vi "2D_Plot.ly_Ex.vi"() -> ()   [LabVIEW 2025]
doc: "Demonstratese how to plot an array with timebase to Plot.ly."
uses:
  <vilib>/Foerster.tech/LabPlot.ly/LabPlot.ly/Typdef/graphSettings.ctl
  <vilib>/Foerster.tech/LabPlot.ly/LabPlot.ly/Typdef/mode.ctl
  <vilib>/Foerster.tech/LabPlot.ly/LabPlot.ly/Typdef/line.ctl
  <vilib>/Foerster.tech/LabPlot.ly/LabPlot.ly/Typdef/dash.ctl
  <vilib>/Analysis/1siggen.llb/Ramp Pattern by Samples.vi
  <vilib>/Analysis/NI_AALBase.lvlib
  <vilib>/Foerster.tech/LabPlot.ly/LabPlot.ly/LabPlot.ly.lvlib
panel:
  out "File Path out":path
  out "Execution Time[ms]":u32
  in  "cycles":dbl=5.0 format="%0.2f"
  in  "Call Setup":bool
  in  "graphSettings":T1={"mode"=enum."lines+markers", "line"={"color"=44543, "width"=2, "dash"=enum."solid"}}
  in  "File Path Control(empty: only show graph)":path
  in  "Reduction(0: No Reduction)":i32
  in  "amplitude":dbl=5.0 format="%0.2f"
  in  "samples":i32=50000
  out "XY Graph":T5(graph)
  # "Sinewave Settings"
  # "Call asynchronously to not hold up your program"
  # "This Program demonstrates how to print a 2D Array consisting of timebase and data to Plot.ly\n\nYou can output the plot to browser without saving it by leaving File Path empty or save the html file by selecting a path.\n\nSince Plot.ly stores the data in the html, plots of >200k points become slow to open. It's recommended you use the built-in Reduction to reduce your dataset."
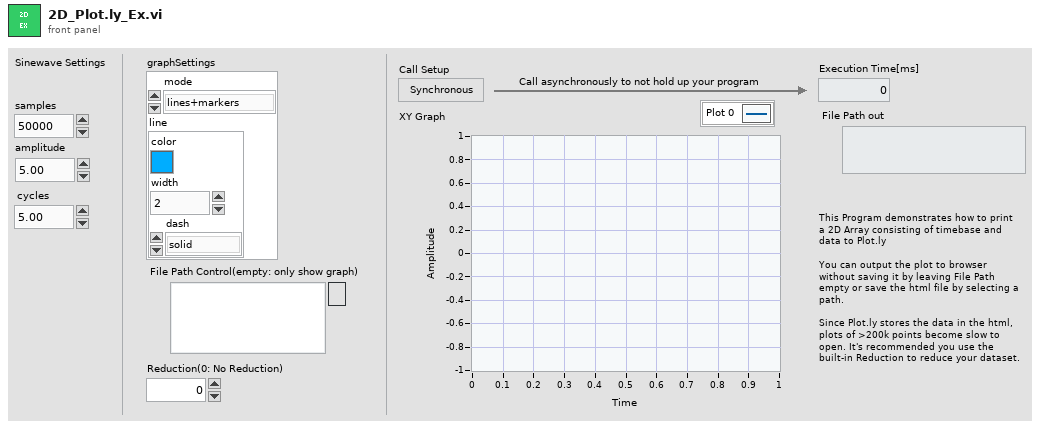
[diagram p1: front panel]
types:
  T1 = typedef "LabPlot.ly.lvlib/graphSettings.ctl" = cluster{"mode":T2, "line":T3}
  T2 = typedef "LabPlot.ly.lvlib/mode.ctl" = enum16{"lines", "markers", "text", "lines+markers", "markers+text", "lines+text", "lines+markers+text"}
  T3 = typedef "LabPlot.ly.lvlib/line.ctl" = cluster{"color":u32, "width":i32, "dash":T4}
  T4 = typedef "LabPlot.ly.lvlib/dash.ctl" = enum16{"solid", "dot", "dash", "longdash", "dashdot", "longdashdot"}
  T5 = cluster{"Ramp Pattern":dbl[], "Sinusoidal Pattern":dbl[]}
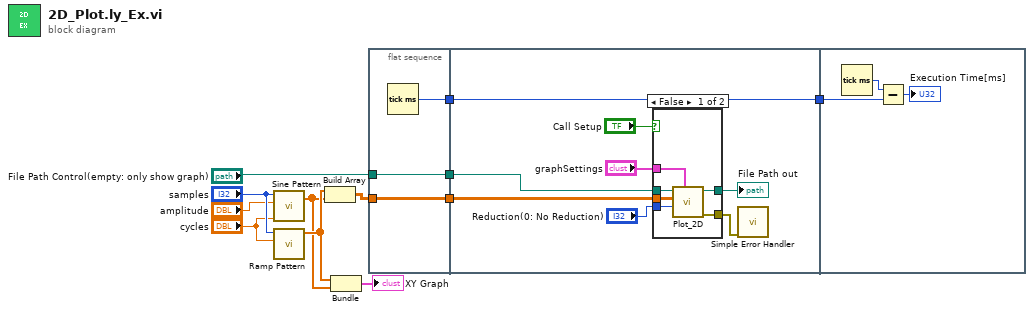
[diagram p0: block diagram]
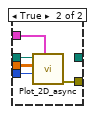
[diagram p2: hidden frame]
diagram:
  n1 = call <vilib>:"Sine Pattern.vi"("cycles"="cycles", "amplitude"="amplitude", "samples"="samples") -> ("Sinusoidal Pattern"=w6:dbl[])  [unwired: 1 in, 1 out]
  n2 = call-poly <vilib>:"Ramp Pattern.vi"("end"="cycles", "samples"="samples") -> ("Ramp Pattern"=w7:dbl[])  [unwired: 8 in, 1 out]
  n3 = Build Array(w7, w6) -> (w8:dbl[][])
  n4 = Bundle("Ramp Pattern"=w7, "Sinusoidal Pattern"=w6) -> (→"XY Graph":T5)  [unwired: 1 in]
  n5 = flat-sequence {
    tunnel: "File Path Control(empty: only show graph)" -> [w15]
    tunnel: [w15] -> w12
    tunnel: [w14] -> w11
    tunnel: w8 -> [w13]
    tunnel: [w13] -> w9
    tunnel: w12 -> [w23]
    tunnel: w11 -> [w22]
    tunnel: [w22] -> w10
    tunnel: w9 -> [w21]
    tunnel: w10 -> [w36]
    frame #0 {
      n6 = Tick Count (ms)() -> (millisecond timer value=w14:u32)
    }
    frame #1 {
      n7 = case shown="False" "Call Setup" {
        tunnel: "Reduction(0: No Reduction)" -> [w29 w32]
        tunnel: w23 -> [w28 w34]
        tunnel: "graphSettings" -> [w24 w33]
        tunnel: [w27 w31] -> w19
        tunnel: [w26 _] -> w20
        tunnel: w21 -> [w25 w30]
        frame False {
          n8 = call <vilib>:"Plot_2D.vi"("graphSettings"=w24, "Reduction(0: No Reduction)"=w29, "1D-Data"=w25, "File Path Control(empty: only show graph)"=w28) -> ("Error Out"=w27:errorcluster, "File Path Indicator"=w26:path)  [unwired: 6 in]
        }
        frame True {
          n9 = call <vilib>:"Plot_2D_async.vi"("graphSettings"=w33, "Reduction(0: No Reduction)"=w32, "1D-Data"=w30, "File Path Control(empty: only show graph)"=w34) -> ("Error Out"=w31:errorcluster)  [unwired: 7 in]
        }
      }
      "File Path out" <- w20
      n10 = call <vilib>:"Simple Error Handler.vi"("error in (no error)"=w19) -> ()  [unwired: 4 in, 5 out]
    }
    frame #2 {
      n11 = Tick Count (ms)() -> (millisecond timer value=w37:u32)
      n12 = Subtract(x=w37, y=w36) -> (x-y=→"Execution Time[ms]":u32)
    }
  }
